vi "Setup subWorker - CPU Percent.vi"(8 "error in":errorcluster, 11 "Controller in":refnum<class "Controller.lvclass">) -> (0 "error out":errorcluster, 3 "Controller out":refnum<class "Controller.lvclass">)   [LabVIEW 2024, in "Controller.lvclass"]
doc: "This VI sets up the framework parameters of a statically-linked subWorker."
uses:
  Controller.lvclass
  Controller.lvclass/Controller.ctl
  CPU Percent/CPU Percent.lvclass
  C:/Program Files (x86)/National Instruments/LabVIEW 2024/vi.lib/addons/_Workers/Library/Classes/Worker/Worker.lvclass
  C:/Program Files (x86)/National Instruments/LabVIEW 2024/vi.lib/addons/_Workers/Library/Classes/Workers Object/Workers Object.lvclass
  C:/_Repo/ugm24-dp2/src/Workers/CPU Percent/CPU Percent.lvclass
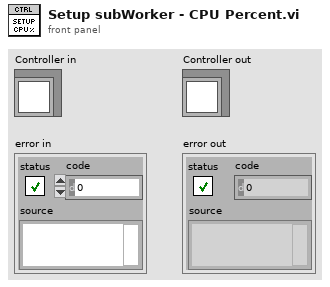
[diagram p1: front panel]
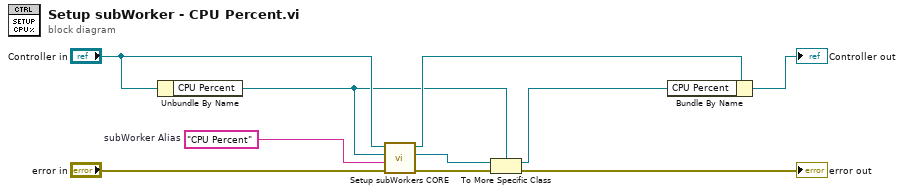
[diagram p0: block diagram]
diagram:
  w6 = "CPU Percent"  # subWorker Alias
  n1 = Unbundle By Name("Controller in") -> ("CPU Percent"=w3:refnum<class "CPU Percent.lvclass">)
  n2 = call-dynamic "Setup subWorkers CORE.vi"("error in"="error in", "subWorker Alias"=w6, "subWorker"=w3, "Worker"="Controller in") -> ("error out"=w5:errorcluster, "subWorker out"=w1:refnum<class "Worker.lvclass">, "Worker out"=w8:refnum<class "Controller.lvclass">)  [unwired: 5 in]
  n3 = To More Specific Class(target class=w3, reference=w1, error in=w5) -> (specific class reference=w2:refnum<class "CPU Percent.lvclass">, error out=→"error out":errorcluster)
  n4 = Bundle By Name(cluster=w8, "CPU Percent"=w2) -> (→"Controller out":refnum<class "Controller.lvclass">)
